vi "Get Distance from Sensor.vi"(2 "Max Distance":dbl, 3 "Distance (m)":fxp<+/-,26,5>, 4 "Sensor Position":T1) -> (0 "In Range?":bool, 1 "Object Position (robot)":cluster{"Object x":dbl, "Object y":dbl})   [LabVIEW 2012]
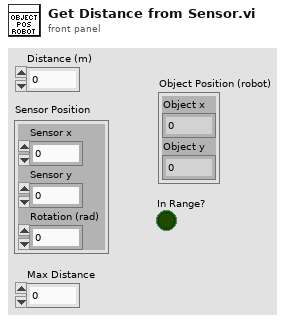
[diagram p1: front panel]
types:
  T1 = cluster{"Sensor x":dbl, "Sensor y":dbl, "Rotation (rad)":dbl}
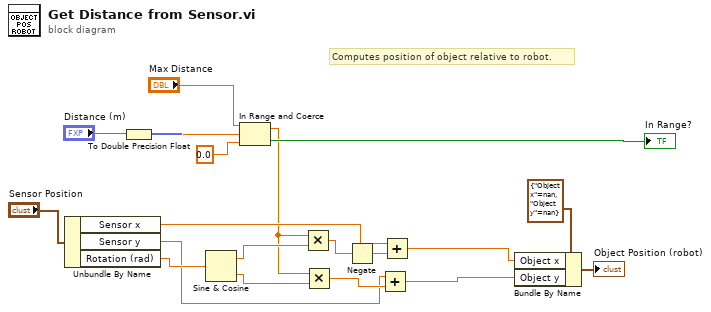
[diagram p0: block diagram]
diagram:
  # "Computes position of object relative to robot."
  n1 = Unbundle By Name("Sensor Position") -> ("Sensor x"=w10:dbl, "Sensor y"=w9:dbl, "Rotation (rad)"=w11:dbl)
  n2 = To Double Precision Float(number="Distance (m)") -> (double precision float=w5:dbl)
  n3 = Sine & Cosine(0:w11) -> (1:w19:dbl, 2:w18:dbl)
  n4 = In Range and Coerce(upper limit="Max Distance", x=w5, lower limit=0.0) -> (coerced(x)=w1:dbl, In Range?=→"In Range?":bool)
  n5 = Multiply(x=w1, y=w19) -> (x*y=w13:dbl)
  n6 = Multiply(x=w1, y=w18) -> (x*y=w12:dbl)
  n7 = Negate(x=w13) -> (-x=w8:dbl)
  n8 = Add(x=w9, y=w12) -> (x+y=w7:dbl)
  n9 = Add(x=w10, y=w8) -> (x+y=w6:dbl)
  n10 = Bundle By Name(cluster=cluster{"Object x":dbl, "Object y":dbl} {"Object x"=nan, "Object y"=nan} ("input cluster"), "Object x"=w6, "Object y"=w7) -> (→"Object Position (robot)":cluster{"Object x":dbl, "Object y":dbl})
